vi "RT_TVAi_r (SubVI).vi"(0 "roll1":dbl, 5 "TVA_p":dbl, 7 "TVA_y":dbl) -> (6 "Act315_Act225":dbl[](array[numeric]))   [LabVIEW 2017]
panel:
  out "Act225":dbl
  out "Act315":dbl
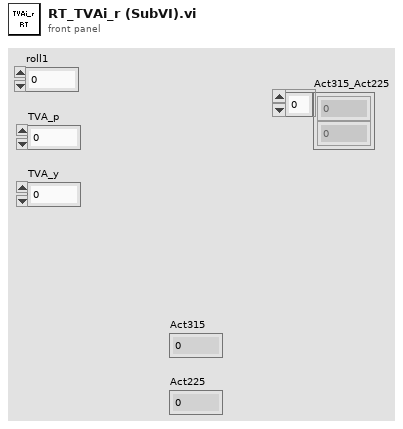
[diagram p1: front panel]
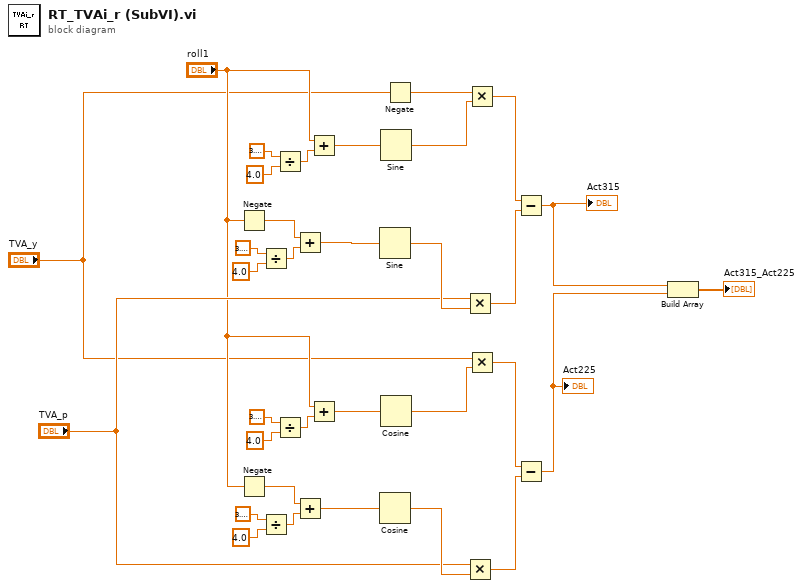
[diagram p0: block diagram]
diagram:
  n1 = Negate(x="roll1") -> (-x=w19:dbl)
  n2 = Negate(x="roll1") -> (-x=w16:dbl)
  n3 = Divide(x=3.141592653589793, y=4.0) -> (x/y=w20:dbl)
  n4 = Divide(x=3.141592653589793, y=4.0) -> (x/y=w15:dbl)
  n5 = Divide(x=3.141592653589793, y=4.0) -> (x/y=w30:dbl)
  n6 = Divide(x=3.141592653589793, y=4.0) -> (x/y=w6:dbl)
  n7 = Add(x=w19, y=w20) -> (x+y=w18:dbl)
  n8 = Add(x=w16, y=w15) -> (x+y=w17:dbl)
  n9 = Add(x="roll1", y=w30) -> (x+y=w31:dbl)
  n10 = Add(x="roll1", y=w6) -> (x+y=w5:dbl)
  n11 = Sine(x=w18) -> (sin(x)=w23:dbl)
  n12 = Cosine(x=w17) -> (cos(x)=w12:dbl)
  n13 = Sine(x=w31) -> (sin(x)=w24:dbl)
  n14 = Cosine(x=w5) -> (cos(x)=w11:dbl)
  n15 = Negate(x="TVA_y") -> (-x=w25:dbl)
  n16 = Multiply(x="TVA_p", y=w23) -> (x*y=w26:dbl)
  n17 = Multiply(x="TVA_p", y=w12) -> (x*y=w10:dbl)
  n18 = Multiply(x=w25, y=w24) -> (x*y=w27:dbl)
  n19 = Multiply(x="TVA_y", y=w11) -> (x*y=w9:dbl)
  n20 = Subtract(x=w27, y=w26) -> (x-y=w32:dbl)
  "Act315" <- w32
  n21 = Subtract(x=w9, y=w10) -> (x-y=w1:dbl)
  "Act225" <- w1
  n22 = Build Array(w32, w1) -> (→"Act315_Act225":dbl[])
